vi "Move Uninitialize VIs into Protected Folder.vi"   [LabVIEW 2015]
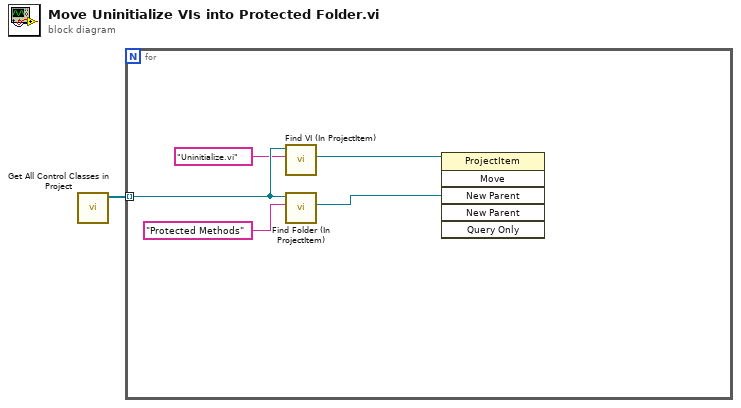
[diagram p0: block diagram]
diagram:
  n1 = call "Get All Control Classes in Project.vi"() -> ("All Control Classes"=w1:refnum<vi>[])  [unwired: 11 in]
  n2 = for {
    tunnel: w1 -> [w6] mode=indexing
    n3 = call "Find VI (In ProjectItem).vi"("VI Name"="Uninitialize.vi", "ProjectItem in"=w6) -> ("VI ProjectItem Refnum"=w3:refnum<vi>)  [unwired: 7 in, 2 out]
    n4 = call "Find Folder (In ProjectItem).vi"("Folder Name"="Protected Methods" ("VI Name"), "ProjectItem in"=w6) -> ("Folder Refnum"=w2:refnum<vi>)  [unwired: 7 in, 2 out]
    n5 = invoke class="ProjectItem" method="Move"(reference=w3, "New Parent"=w2) -> ()  [unwired: 4 in, 6 out]
  }
